vi "Set Generation Type.vi"(7 "Generation Type":T1, 8 "error in (no error)":errorcluster, 11 "Message Channel in":T2 format="%.0x") -> (0 "error out":errorcluster, 3 "Item Ref out":T2 format="%.0x")   [LabVIEW 2018, in "Instrument Addon Scripting API.lvlib"]
uses:
  Instrument Addon Scripting API.lvlib
  <vilib>/NI Veristand/Custom Device API/Custom Device Item Ref.ctl
  Addon/Addon Shared/Types/Message Generation Type.ctl
  Addon/Addon Shared/Types/FG Control.ctl
  Addon/Addon Shared/SubVIs/Constants.vi
  <vilib>/NI Veristand/Custom Device API/NI VeriStand - Get Item Property.vi
  <vilib>/NI Veristand/Custom Device API/Get Item Property (U32).vi
  <vilib>/NI Veristand/Custom Device API/Get Item Property (Double).vi
  <vilib>/NI Veristand/Custom Device API/Get Item Property (Boolean).vi
  <vilib>/NI Veristand/Custom Device API/Get Item Property (String).vi
  <vilib>/NI Veristand/Custom Device API/NI VeriStand - Set Item Property.vi
  <vilib>/NI Veristand/Custom Device API/Set Item Property (U32).vi
  <vilib>/NI Veristand/Custom Device API/Set Item Property (Double).vi
  <vilib>/NI Veristand/Custom Device API/Set Item Property (Boolean).vi
  <vilib>/NI Veristand/Custom Device API/Set Item Property (String).vi
  Addon/Addon Shared/Instrument Addon Shared.lvlib
  <vilib>/NI Veristand/Custom Device API/Custom Device API.lvlib
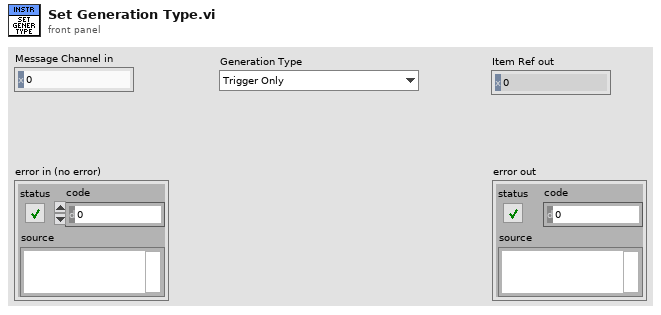
[diagram p1: front panel]
types:
  T1 = typedef "Instrument Addon Shared.lvlib/Message Generation Type.ctl" = enum16{"Trigger Only", "Periodic & Trigger", "Value Change & Trigger"}
  T2 = typedef "Custom Device API.lvlib/Custom Device Item Ref.ctl" = u64
  T3 = typedef "Instrument Addon Shared.lvlib/FG Control.ctl" = enum16{"Get", "Set"}
  T4 = typedef "Instrument Addon Shared.lvlib/Message Parameters.ctl" = cluster{"Generation Type":T1, "Period":dbl, "Include Protection":bool, "Type":string}
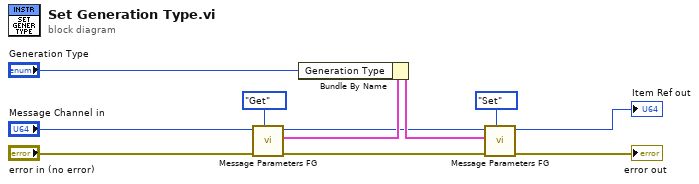
[diagram p0: block diagram]
diagram:
  n1 = call "Message Parameters FG.vi"("Action"=FG_Control."Get", "error in (no error)"="error in (no error)", "Item Ref in"="Message Channel in") -> ("error out"=w1:errorcluster, "Message Settings out"=w4:T4, "Item Ref out"=w2:T2)  [unwired: 6 in]
  n2 = Bundle By Name(cluster=w4, "Generation Type"="Generation Type") -> (w5:T4)
  n3 = call "Message Parameters FG.vi"("Action"=FG_Control."Set", "error in (no error)"=w1, "Message Settings"=w5, "Item Ref in"=w2) -> ("error out"=→"error out":errorcluster, "Item Ref out"=→"Item Ref out":T2)  [unwired: 5 in, 1 out]
